vi "RingStringFromValue.vi"(9 "error in (no error)":errorcluster, 10 "SearchValue":dbl, 11 "RingRefin":refnum<vi>) -> (1 "error IO":errorcluster, 3 "StringOut":string)   [LabVIEW 2020]
panel:
  out "Found":bool
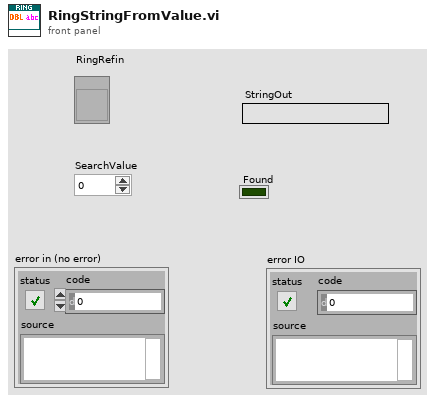
[diagram p1: front panel]
types:
  T1 = typedef "LVStringsAndValuesArrayTypeDef.ctl" = cluster{"String":string, "Value":ext}[]
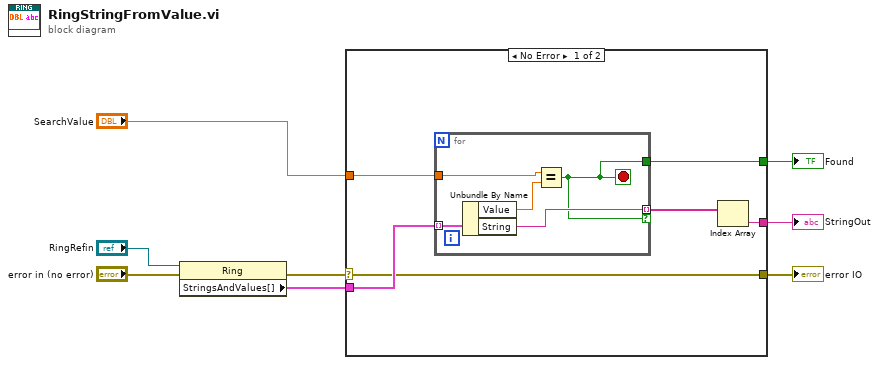
[diagram p0: block diagram]
diagram:
  n1 = property class="Ring"(reference="RingRefin", error in="error in (no error)") -> (error out=w2:errorcluster, "StringsAndValues[]"=w6:T1)  [unwired: 1 out]
  n2 = case shown="No Error" w2 {
    selector: w2 -> [w9 w20]
    tunnel: [w14 _] -> w8
    tunnel: "SearchValue" -> [w12 _]
    tunnel: w6 -> [w11 _]
    tunnel: [w10 _] -> w4
    tunnel: [w9 w20] -> w1
    frame No Error {
      n3 = for {
        tunnel: w11 -> [w19] mode=indexing
        tunnel: [w16] -> w13 mode=indexing if=w15
        tunnel: w12 -> [w17]
        tunnel: [w15] -> w10
        stop <- w15 stop-if-true
        n4 = Unbundle By Name(w19) -> ("Value"=w18:ext, "String"=w16:string)
        n5 = Equal?(x=w17, y=w18) -> (x = y?=w15:bool)
      }
      n6 = Index Array(array=w13) -> (element=w14:string)  [unwired: 1 in]
    }
    frame Error {
    }
  }
  "StringOut" <- w8
  "Found" <- w4
  "error IO" <- w1
